vi "Launcher Calc.vi"() -> ()   [LabVIEW 2020]
uses:
  Calculadora/Calculadora.lvclass
  C:/Program Files (x86)/National Instruments/LabVIEW 2020/vi.lib/ActorFramework/Actor/Actor.lvclass
  Calculadora Messages/Set Numero A Msg/Set Numero A Msg.lvclass/Set Numero A Msg.ctl
  <vilib>/ActorFramework/Message Enqueuer/Message Enqueuer.lvclass/Message Enqueuer.ctl
  Calculadora Messages/Set Numero B Msg/Set Numero B Msg.lvclass/Set Numero B Msg.ctl
  <vilib>/ActorFramework/Message Enqueuer/Enqueue.vi
  Calculadora Messages/Set Numero A Msg/Set Numero A Msg.lvclass
  C:/Program Files (x86)/National Instruments/LabVIEW 2020/vi.lib/ActorFramework/Message/Message.lvclass
  Calculadora Messages/Set Numero B Msg/Set Numero B Msg.lvclass
  <vilib>/ActorFramework/Stop Msg/Stop Msg.lvclass
  Calculadora Messages/Suma Msg/Suma Msg.lvclass
  Calculadora Messages/Resta Msg/Resta Msg.lvclass
  Calculadora Messages/Multiplicacion Msg/Multiplicacion Msg.lvclass
  Calculadora Messages/Division Msg/Division Msg.lvclass
  <vilib>/ActorFramework/Message Priority Queue/Priority Enqueue.vi
  <vilib>/ActorFramework/Actor/Actor.lvclass
  D:/Storage/Source Code/Clase AF/ClaseAF/02 QMH/Calculadora/Calculadora/Calculadora.lvclass
panel:
  in  "Division":bool
  in  "Multiplicacion":bool
  in  "Resta":bool
  in  "Suma":bool
  in  "Stop":bool
  in  "B":dbl(slide) scale=0.0..10.0
  in  "A":dbl(slide) scale=0.0..10.0
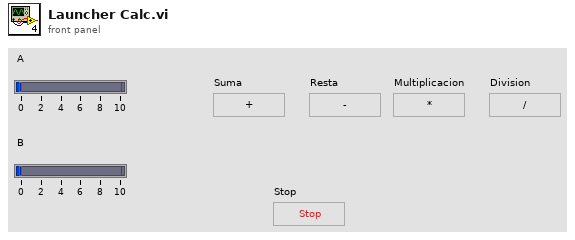
[diagram p1: front panel]
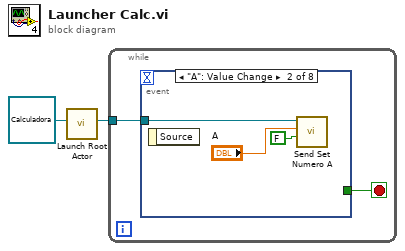
[diagram p0: block diagram]
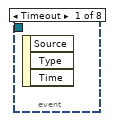
[diagram p2: hidden frame]
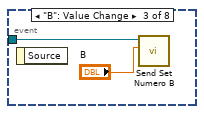
[diagram p3: hidden frame]
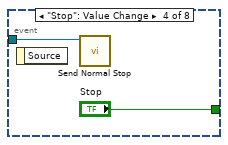
[diagram p4: hidden frame]
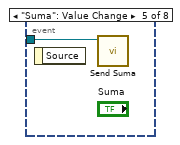
[diagram p5: hidden frame]
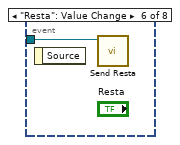
[diagram p6: hidden frame]
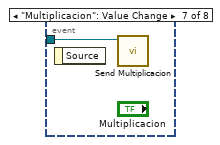
[diagram p7: hidden frame]
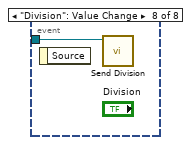
[diagram p8: hidden frame]
diagram:
  n1 = call <vilib>:"Launch Root Actor.vi"("Actor"=refnum<class "Calculadora.lvclass"> refnum ("Calculadora.lvlib:Calculadora.lvclass")) -> ("Actor's Enqueuer"=w1:refnum<class "Message Enqueuer.lvclass">)  [unwired: 9 in, 1 out]
  n2 = while {
    tunnel: w1 -> [w4]
    stop <- w3 stop-if-true
    n3 = event shown="[1] \"A\": Value Change" {
      selector: _ -> [_ _ _ _ _ _ _ _]
      dyn-events: _ -> [_ _ _ _ _ _ _ _]
      timeout: _ -> [_ _ _ _ _ _ _ _]
      tunnel: w4 -> [_ w7 w8 w11 w12 w13 w14 w15]
      tunnel: [_ _ _ "Stop" _ _ _ _] -> w3
      event Timeout {
        n4 = event-data() -> ()  [unwired: 1 in, 3 out]
      }
      event "A": Value Change {
        n5 = event-data() -> ()  [unwired: 1 in, 1 out]
        n6 = call "Send Set Numero A.vi"("Boolean"=FALSE, "Numero A"="A", "Message Enqueuer"=w7) -> ()  [unwired: 7 in, 2 out]
      }
      event "B": Value Change {
        n7 = event-data() -> ()  [unwired: 1 in, 1 out]
        n8 = call "Send Set Numero B.vi"("Numero B"="B", "Message Enqueuer"=w8) -> ()  [unwired: 8 in, 2 out]
      }
      event "Stop": Value Change {
        n9 = event-data() -> ()  [unwired: 1 in, 1 out]
        n10 = call <vilib>:"Send Normal Stop.vi"("Message Enqueuer"=w11) -> ()  [unwired: 10 in, 1 out]
      }
      event "Suma": Value Change {
        n11 = event-data() -> ()  [unwired: 1 in, 1 out]
        n12 = call "Send Suma.vi"("Message Enqueuer"=w12) -> ()  [unwired: 9 in, 2 out]
      }
      event "Resta": Value Change {
        n13 = event-data() -> ()  [unwired: 1 in, 1 out]
        n14 = call "Send Resta.vi"("Message Enqueuer"=w13) -> ()  [unwired: 9 in, 2 out]
      }
      event "Multiplicacion": Value Change {
        n15 = event-data() -> ()  [unwired: 1 in, 1 out]
        n16 = call "Send Multiplicacion.vi"("Message Enqueuer"=w14) -> ()  [unwired: 9 in, 2 out]
      }
      event "Division": Value Change {
        n17 = event-data() -> ()  [unwired: 1 in, 1 out]
        n18 = call "Send Division.vi"("Message Enqueuer"=w15) -> ()  [unwired: 9 in, 2 out]
      }
    }
  }
